vi "Create.vi"(7 "Alpha":dbl, 8 "error in (no error)":errorcluster, 9 "Image Size":T1, 11 "Camera Parameters in":T3) -> (0 "error out":errorcluster, 1 "Valid Pixels Size":T1, 2 "Camera Parameters":T3, 3 "Image Undistorter":refnum<class "Image Undistorter.lvclass">, 5 "Valid Pixels Top Left":T2)   [LabVIEW 2020, in "image.lvlib" / "Image Undistorter.lvclass"]
doc: "Create an Image Undistorter."
uses:
  Image Undistorter.lvclass
  common/Camera Parameters.ctl
  common/Camera Matrix.ctl
  common/Camera Distortion Coefficients.ctl
  common/Image Size (Integer).ctl
  common/Image Point (Integer).ctl
  Image Undistorter.lvclass/Image Undistorter.ctl
  common/common.lvlib
  common/bin/gartoolkit_32-1.dll
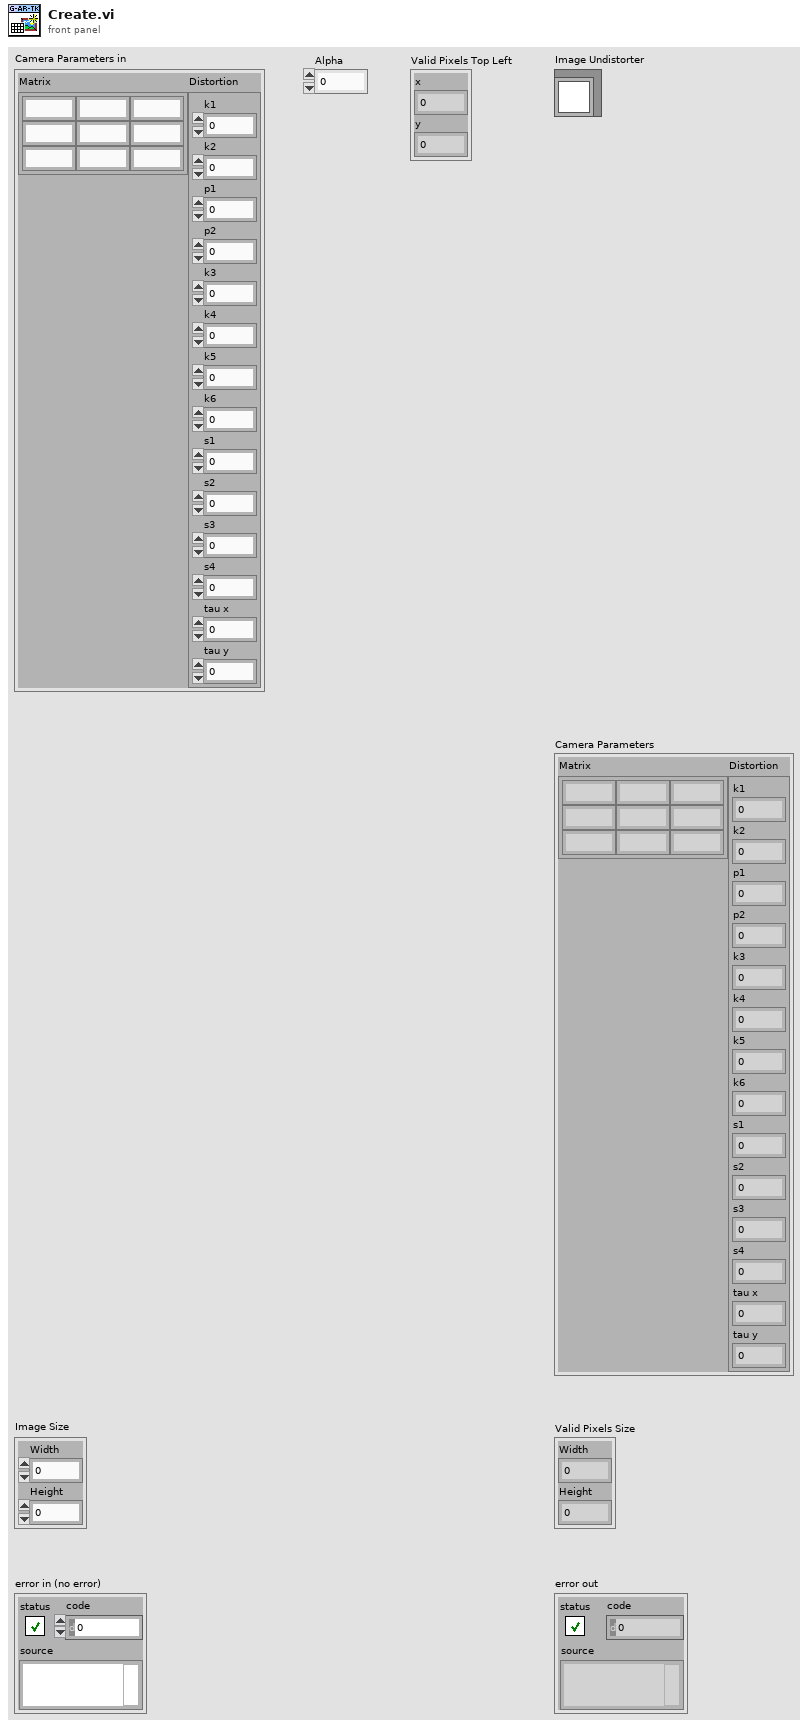
[diagram p1: front panel]
types:
  T1 = typedef "common.lvlib/Image Size (Integer).ctl" = cluster{"Width":u16, "Height":u16}
  T2 = typedef "common.lvlib/Image Point (Integer).ctl" = cluster{"x":i32, "y":i32}
  T3 = typedef "common.lvlib/Camera Parameters.ctl" = cluster{"Matrix":T4, "Distortion":T5}
  T4 = typedef "common.lvlib/Camera Matrix.ctl" = cluster{"m 0,0":dbl, "m 0,1":dbl, "m 0,2":dbl, "m 1,0":dbl, "m 1,1":dbl, "m 1,2":dbl, "m 2,0":dbl, "m 2,1":dbl, "m 2,2":dbl}
  T5 = typedef "common.lvlib/Camera Distortion Coefficients.ctl" = cluster{"k1":dbl, "k2":dbl, "p1":dbl, "p2":dbl, "k3":dbl, "k4":dbl, "k5":dbl, "k6":dbl, "s1":dbl, "s2":dbl, "s3":dbl, "s4":dbl, "tau x":dbl, "tau y":dbl}
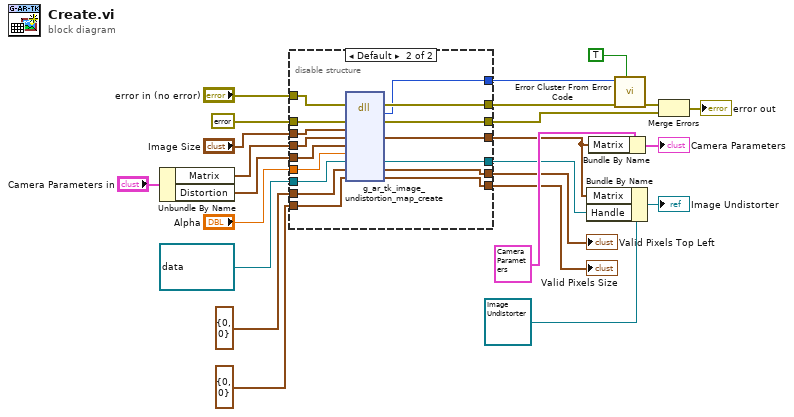
[diagram p0: block diagram]
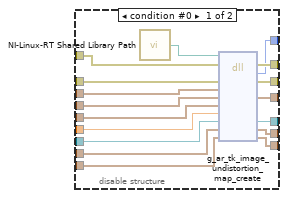
[diagram p2: hidden frame]
diagram:
  n1 = Unbundle By Name("Camera Parameters in") -> ("Matrix"=w14:T4, "Distortion"=w13:T5)
  n2 = disable-structure shown="Default" {
    disable-tunnel: "error in (no error)" -> [w41 w57]
    disable-tunnel: errorcluster {"status"=FALSE, "code"=0, "source"=""} ("error constant") -> [w40 w56]
    disable-tunnel: "Image Size" -> [w39 w55]
    disable-tunnel: w14 -> [w38 w54]
    disable-tunnel: w13 -> [w37 w53]
    disable-tunnel: "Alpha" -> [w36 w52]
    disable-tunnel: refnum<data-value> refnum ("EDVR") -> [w35 w51]
    disable-tunnel: T2 {"x"=0, "y"=0} ("Image Point") -> [w34 w50]
    disable-tunnel: T1 {"Width"=0, "Height"=0} ("roi_bottom_right") -> [w33 w49]
    disable-tunnel: [w32 w48] -> w8
    disable-tunnel: [w31 w47] -> w7
    disable-tunnel: [w30 w46] -> w6
    disable-tunnel: [w29 w45] -> w5
    disable-tunnel: [w28 w44] -> w4
    disable-tunnel: [w27 w43] -> w3
    disable-tunnel: [w26 w42] -> w2
    frame condition #0 {
      n3 = call "NI-Linux-RT Shared Library Path.vi"() -> ("Path"=w25:path)
      n4 = dll-call lib="?" fn="g_ar_tk_image_undistortion_map_create" ("g_ar_toolkit.*.*:g_ar_tk_image_add_weighted")(path in=w25, error in=w41, "error_cluster"=w40, "size"=w39, "camera_matrix"=w38, "distortion_param"=w37, "alpha"=w36, "EDVR"=w35, "roi_top_left"=w34, "roi_size"=w33) -> (error out=w32:errorcluster, w31:i32, "error_cluster"=w30:errorcluster, "camera_matrix"=w29:T4, "EDVR"=w28:refnum<data-value>, "roi_top_left"=w27:T2, "roi_size"=w26:T1)  [unwired: 4 in, 1 out]
    }
    frame condition #1 (active) {
      n5 = dll-call lib="C:/serenial/lib/g-augmented-reality-toolkit/LabVIEW/common/bin/gartoolkit_*-1.*" fn="g_ar_tk_image_undistortion_map_create" ("g_ar_toolkit.*.*:g_ar_tk_image_add_weighted")(error in=w57, "error_cluster"=w56, "size"=w55, "camera_matrix"=w54, "distortion_param"=w53, "alpha"=w52, "EDVR"=w51, "roi_top_left"=w50, "roi_size"=w49) -> (error out=w48:errorcluster, w47:i32, "error_cluster"=w46:errorcluster, "camera_matrix"=w45:T4, "EDVR"=w44:refnum<data-value>, "roi_top_left"=w43:T2, "roi_size"=w42:T1)  [unwired: 5 in, 1 out]
    }
  }
  "Valid Pixels Top Left" <- w3
  "Valid Pixels Size" <- w2
  n6 = Bundle By Name(cluster=refnum<class "Image Undistorter.lvclass"> refnum ("Image Rectifier out"), "Matrix"=w5, "Handle"=w4) -> (→"Image Undistorter":refnum<class "Image Undistorter.lvclass">)
  n7 = Bundle By Name(cluster=T3 {"Matrix"={"m 0,0"=0.0, "m 0,1"=0.0, "m 0,2"=0.0, "m 1,0"=0.0, "m 1,1"=0.0, "m 1,2"=0.0, "m 2,0"=0.0, "m 2,1"=0.0, "m 2,2"=0.0}, "Distortion"={"k1"=0.0, "k2"=0.0, "p1"=0.0, "p2"=0.0, "k3"=0.0, "k4"=0.0, "k5"=0.0, "k6"=0.0, "s1"=0.0, "s2"=0.0, "s3"=0.0, "s4"=0.0, "tau x"=0.0, "tau y"=0.0}} ("Camera Parameters in"), "Matrix"=w5) -> (→"Camera Parameters":T3)
  n8 = call <vilib>:"Error Cluster From Error Code.vi"("show call chain? (False)"=TRUE, "error in (no error)"=w8, "error code (0)"=w7) -> ("error out"=w24:errorcluster)  [unwired: 6 in]
  n9 = Merge Errors(w24, w6) -> (→"error out":errorcluster)
